vi "Drive Straight.vi"(10 "Angle robot facing":dbl, 11 "drive.lvclass":refnum<class "drive.lvclass">) -> (2 "Arcade drive x":dbl, 3 "drive.lvclass":refnum<class "drive.lvclass">)   [LabVIEW 2015, in "drive.lvclass"]
uses:
  drive.lvclass
  <vilib>/addons/control/pid/pid.llb/PID (DBL).vi
  <vilib>/addons/control/pid/NI_PID_pid.lvlib
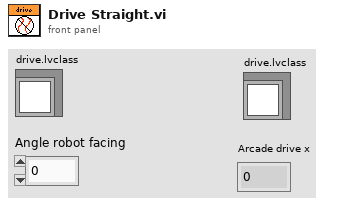
[diagram p1: front panel]
types:
  T1 = cluster{"proportional gain (Kc)":dbl, "integral time (Ti, min)":dbl, "derivative time (Td, min)":dbl}
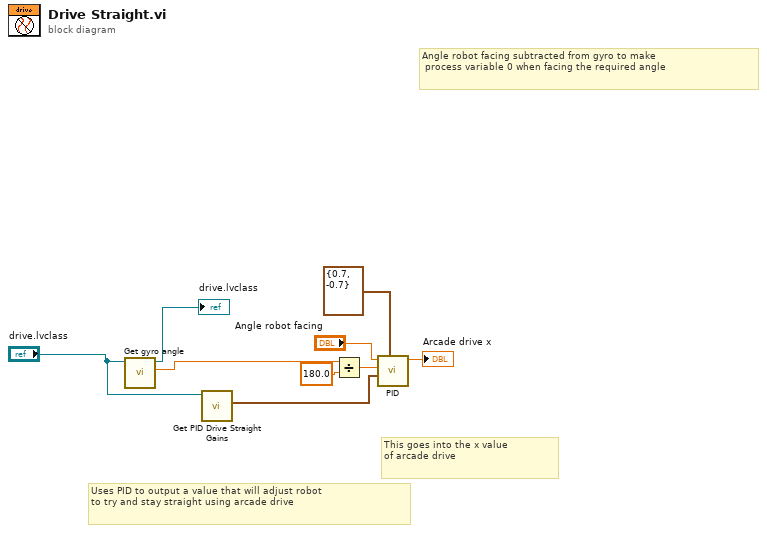
[diagram p0: block diagram]
diagram:
  # "This goes into the x value \nof arcade drive"
  # "Angle robot facing subtracted from gyro to make\n process variable 0 when facing the required angle"
  # "Uses PID to output a value that will adjust robot\nto try and stay straight using arcade drive"
  n1 = call "Get gyro angle.vi"("drive in"="drive.lvclass") -> ("Angle"=w4:dbl, "drive out"=→"drive.lvclass":refnum<class "drive.lvclass">)  [unwired: 9 in]
  n2 = call "Get PID Drive Straight Gains.vi"("drive in"="drive.lvclass") -> ("PID Drive Straight Gains"=w3:T1)  [unwired: 9 in, 1 out]
  n3 = Divide(x=w4, y=180.0) -> (x/y=w8:dbl)
  n4 = call-poly <vilib>:"PID.vi"("output range"=cluster{"output high":dbl, "output low":dbl} {"output high"=0.7, "output low"=-0.7}, "PID gains"=w3, "process variable"=w8, "setpoint"="Angle robot facing") -> ("output"=→"Arcade drive x":dbl)  [unwired: 6 in, 1 out]
